vi "Sort.vi"(8 "error in (no error)":errorcluster, 11 "Array in":string[][](array[string])) -> (0 "error out":errorcluster, 3 "Array out":string[][](array[string]))   [LabVIEW 2015, in "Project.lvclass"]
uses:
  Project.lvclass
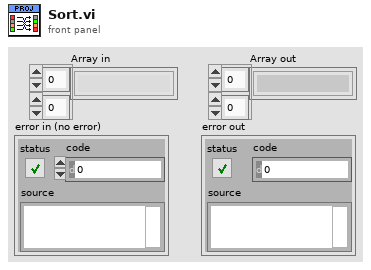
[diagram p1: front panel]
types:
  T1 = typedef "Project.lvclass/FPGA Settings.ctl" = cluster{"FPGA Target Name":string, "Modules":T2[]}
  T2 = typedef "Module.lvclass/Module Settings.ctl" = cluster{"Group Name":string, "Model Number":string, "Signals":T3[]}
  T3 = typedef "Signal.lvclass/Signal Settings.ctl" = cluster{"Signal Name":string, "IO Name":string, "Signal Type":string, "Signal Parameters":string, "IO Resource":string}
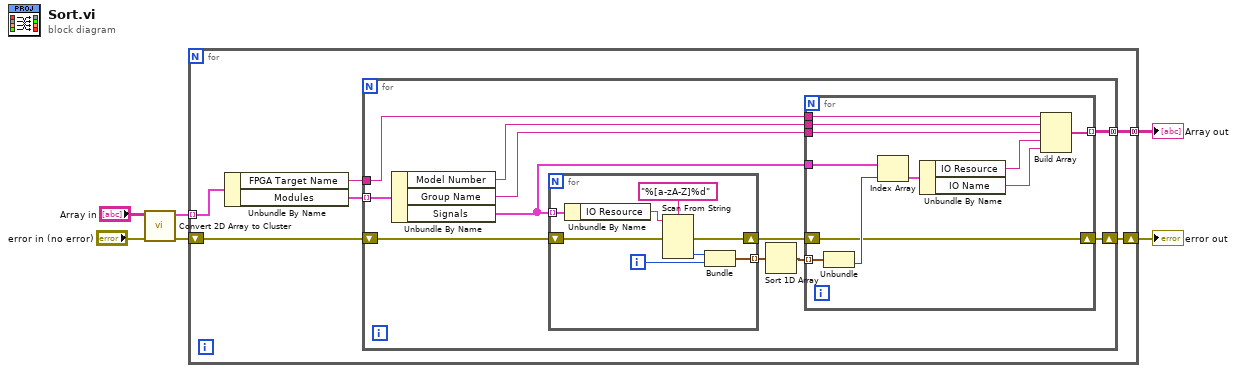
[diagram p0: block diagram]
diagram:
  n1 = call "Convert 2D Array to Cluster.vi"("error in (no error)"="error in (no error)", "Array in"="Array in") -> ("error out"=w3:errorcluster, "Array out"=w5:T1[])  [unwired: 8 in]
  n2 = for {
    tunnel: w5 -> [w10] mode=indexing
    shift-right: [w9] -> w1
    shift-left: w3 -> [w11]
    tunnel: [w7] -> w2 mode=concatenating
    n3 = Unbundle By Name(w10) -> ("FPGA Target Name"=w8:string, "Modules"=w12:T2[])
    n4 = for {
      tunnel: w12 -> [w18] mode=indexing
      shift-right: [w17] -> w9
      shift-left: w11 -> [w20]
      tunnel: w8 -> [w16]
      tunnel: [w13] -> w7 mode=concatenating
      n5 = Unbundle By Name(w18) -> ("Model Number"=w15:string, "Group Name"=w14:string, "Signals"=w21:T3[])
      n6 = for {
        tunnel: w21 -> [w42] mode=indexing
        tunnel: [w37] -> w23 mode=indexing
        shift-right: [w35] -> w19
        shift-left: w20 -> [w36]
        i -> [w38]
        n7 = Unbundle By Name(w42) -> ("IO Resource"=w40:string)
        n8 = Scan From String(format string="%[a-zA-Z]%d", input string=w40, error in=w36) -> (error out=w35:errorcluster, output 2=w39:i32)  [unwired: 4 in, 2 out]
        n9 = Bundle(w39, w38) -> (w37:cluster{i32, i32})  [unwired: 1 in]
      }
      n10 = Sort 1D Array(array=w23) -> (sorted array=w22:cluster{i32, i32}[])
      n11 = for {
        tunnel: w22 -> [w34] mode=indexing
        tunnel: w21 -> [w32]
        shift-right: [w30] -> w17
        shift-left: w19 -> [w30]
        tunnel: w16 -> [w29]
        tunnel: w15 -> [w28]
        tunnel: w14 -> [w27]
        tunnel: [w24] -> w13 mode=indexing
        n12 = Unbundle(w34) -> (w33:i32)  [unwired: 1 out]
        n13 = Index Array(array=w32, index=w33) -> (element=w31:T3)
        n14 = Unbundle By Name(w31) -> ("IO Resource"=w26:string, "IO Name"=w25:string)
        n15 = Build Array(w29, w28, w27, w26, w25) -> (w24:string[])
      }
    }
  }
  "Array out" <- w2
  "error out" <- w1
